vi "TestAFM_Driver_Manager.vi"() -> ()   [LabVIEW 2019]
uses:
  lvsrc/subVIs/AFM API/AFM_Driver_Manager/AFM_Driver_Manager.lvclass
  <vilib>/addons/_JKI Toolkits/Caraya/classes/Test/Test.lvclass
  <vilib>/addons/_JKI Toolkits/Caraya/classes/Assert/Assert.lvclass
  <vilib>/addons/_JKI Toolkits/Caraya/classes/Assert/Assert Equal Value_Variant.vi
  <userlib>/LevyLab/Relay Box/Typedefs/Resistor--enum.ctl
  <vilib>/addons/_JKI Toolkits/Caraya/classes/Assert/Assert True.vi
  <vilib>/addons/_JKI Toolkits/Caraya/classes/Assert/Assert Not Error.vi
panel:
  in  "error in (no error)":errorcluster
  out "error out":errorcluster
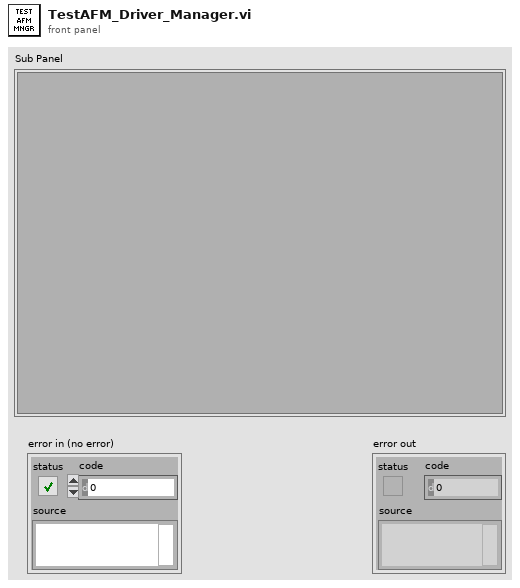
[diagram p1: front panel]
types:
  T1 = typedef "Resistor--enum.ctl" = enum16{"open", "discharge tip", "0 ohms", "100k ohm", "10M ohm", "1G ohm"}
  T2 = cluster{"Name":string, "Litho":cluster{"X":dbl, "Y":dbl, "Speed":dbl, "Voltage":dbl}[], "Set Resistance":T1, "Meta":variant}[]
  T3 = typedef "AFM_Driver_Manager.lvclass/AFM_Driver_Manager.PublicMethods.ctl" = cluster{"Stop Event":refnum<user-event>, "Lithography Data":refnum<user-event>, "Run Lithography":refnum<user-event>, "Background Image":refnum<user-event>, "Abort Notifier":refnum<user-event>}
  T4 = cluster{"VI Refnum":refnum<vi>, "Path":path, "Name":string, "Events":T3}
  T5 = typedef "AFM_Driver_Manager.lvclass/AFM_Driver_Manager.PublicEvents.ctl" = cluster{"Lithography Done":refnum<user-event>}
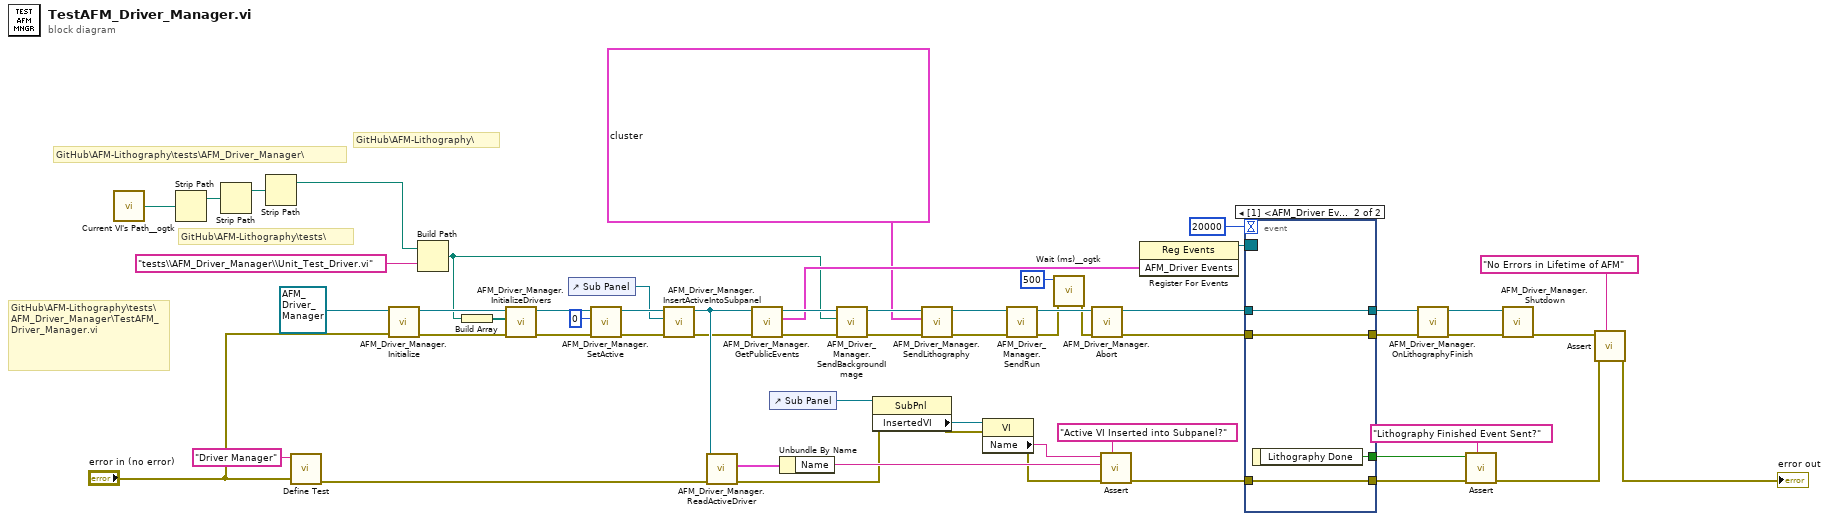
[diagram p0: block diagram]
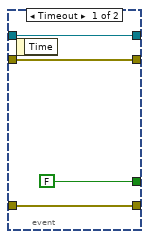
[diagram p2: hidden frame]
diagram:
  # "GitHub\\AFM-Lithography\\tests\\"
  # "GitHub\\AFM-Lithography\\tests\\AFM_Driver_Manager\\"
  # "GitHub\\AFM-Lithography\\"
  # "GitHub\\AFM-Lithography\\tests\\AFM_Driver_Manager\\TestAFM_Driver_Manager.vi"
  n1 = call <userlib>:"Current VI's Path__ogtk.vi"() -> ("Current VI's Path (+ Relative)"=w58:path)  [unwired: 1 in]
  n2 = Strip Path(path=w58) -> (stripped path=w57:path)  [unwired: 1 out]
  n3 = Strip Path(path=w57) -> (stripped path=w56:path)  [unwired: 1 out]
  n4 = Strip Path(path=w56) -> (stripped path=w1:path)  [unwired: 1 out]
  n5 = call <vilib>:"Define Test.vi"("error in (no error)"="error in (no error)", "Label (VI Title)"="Driver Manager") -> ("error out"=w24:errorcluster)  [unwired: 9 in]
  n6 = call "AFM_Driver_Manager.Initialize.vi"("error in (no error)"="error in (no error)", "AFM_Driver_Manager in"=refnum<class "AFM_Driver_Manager.lvclass"> refnum) -> ("error out"=w34:errorcluster, "AFM_Driver_Manager out"=w54:refnum<class "AFM_Driver_Manager.lvclass">)  [unwired: 8 in]
  n7 = Build Path(base path=w1, name or relative path="tests\\AFM_Driver_Manager\\Unit_Test_Driver.vi") -> (appended path=w10:path)
  n8 = Build Array(w10) -> (w31:path[])
  n9 = call "AFM_Driver_Manager.InitializeDrivers.vi"("error in (no error)"=w34, "Paths"=w31, "AFM_Driver_Manager in"=w54) -> ("error out"=w33:errorcluster, "AFM_Driver_Manager out"=w53:refnum<class "AFM_Driver_Manager.lvclass">)  [unwired: 7 in]
  n10 = control-ref of="Sub Panel"() -> (w27:refnum<vi>)
  n11 = call "AFM_Driver_Manager.SetActive.vi"("error in (no error)"=w33, "Active Index"=0, "AFM_Driver_Manager in"=w53) -> ("error out"=w32:errorcluster, "AFM_Driver_Manager out"=w52:refnum<class "AFM_Driver_Manager.lvclass">)  [unwired: 7 in]
  n12 = call "AFM_Driver_Manager.InsertActiveIntoSubpanel.vi"("error in (no error)"=w32, "SubPnl Refnum"=w27, "AFM_Driver_Manager in"=w52) -> ("error out"=w15:errorcluster, "AFM_Driver_Manager out"=w26:refnum<class "AFM_Driver_Manager.lvclass">)  [unwired: 7 in]
  n13 = call "AFM_Driver_Manager.ReadActiveDriver.vi"("error in (no error)"=w24, "AFM_Driver_Manager in"=w26) -> ("error out"=w22:errorcluster, "Active Driver"=w25:T4)  [unwired: 7 in, 1 out]
  n14 = call "AFM_Driver_Manager.GetPublicEvents.vi"("error in (no error)"=w15, "AFM_Driver_Manager in"=w26) -> ("error out"=w49:errorcluster, "AFM_Driver Events"=w35:T5, "AFM_Driver_Manager out"=w50:refnum<class "AFM_Driver_Manager.lvclass">)  [unwired: 7 in]
  n15 = control-ref of="Sub Panel"() -> (w17:refnum<vi>)
  n16 = Unbundle By Name(w25) -> ("Name"=w23:string)
  n17 = call "AFM_Driver_Manager.SendBackgroundImage.vi"("error in (no error)"=w49, "Path"=w10, "AFM_Driver_Manager in"=w50) -> ("error out"=w47:errorcluster, "AFM_Driver_Manager out"=w48:refnum<class "AFM_Driver_Manager.lvclass">)  [unwired: 7 in]
  n18 = property class="SubPnl"(reference=w17, error in=w22) -> (error out=w14:errorcluster, "InsertedVI"=w16:refnum<vi>)  [unwired: 1 out]
  n19 = call "AFM_Driver_Manager.SendLithography.vi"("error in (no error)"=w47, "Lithography Data"=T2 [{"Name"="p0", "Litho"=[{"X"=1.0, "Y"=2.0, "Speed"=3.0, "Voltage"=4.0}], "Set Resistance"=enum."discharge tip", "Meta"=variant}, {"Name"="p1", "Litho"=[{"X"=5.0, "Y"=6.0, "Speed"=7.0, "Voltage"=8.0}], "Set Resistance"=enum."open", "Meta"=variant}], "AFM_Driver_Manager in"=w48) -> ("error out"=w45:errorcluster, "AFM_Driver_Manager out"=w46:refnum<class "AFM_Driver_Manager.lvclass">)  [unwired: 7 in]
  n20 = property class="VI"(reference=w16, error in=w14) -> (error out=w13:errorcluster, "Name"=w12:string)  [unwired: 1 out]
  n21 = call "AFM_Driver_Manager.SendRun.vi"("error in (no error)"=w45, "AFM_Driver_Manager in"=w46) -> ("error out"=w8:errorcluster, "AFM_Driver_Manager out"=w44:refnum<class "AFM_Driver_Manager.lvclass">)  [unwired: 8 in]
  n22 = call <userlib>:"Wait (ms)__ogtk.vi"("error in (no error)"=w8, "milliseconds to wait"=u32 500) -> ("error out"=w9:errorcluster)  [unwired: 8 in, 1 out]
  n23 = call "AFM_Driver_Manager.Abort.vi"("error in (no error)"=w9, "AFM_Driver_Manager in"=w44) -> ("error out"=w38:errorcluster, "AFM_Driver_Manager out"=w40:refnum<class "AFM_Driver_Manager.lvclass">)  [unwired: 8 in]
  n24 = call-poly <vilib>:"Assert.vi"("Label"="Active VI Inserted into Subpanel?" ("Label (VI Title)"), "error in (no error)"=w13, "Y"=w23, "X"=w12) -> ("error out"=w20:errorcluster)  [unwired: 7 in]
  n25 = register-events(w35) -> (reference out=w36:refnum<event-registration>)  [unwired: 2 in, 1 out]
  n26 = event shown="[1] <AFM_Driver Events.Lithography Done>: User Event" {
    selector: w36 -> [_ _]
    dyn-events: _ -> [_ _]
    timeout: 20000 -> [_ _]
    tunnel: [w62 w66] -> w41
    tunnel: w40 -> [w62 w66]
    tunnel: [w61 w65] -> w39
    tunnel: w38 -> [w61 w65]
    tunnel: [FALSE w64] -> w21
    tunnel: w20 -> [w60 w63]
    tunnel: [w60 w63] -> w19
    event Timeout {
      n27 = event-data() -> ()  [unwired: 1 in, 1 out]
    }
    event User Event {
      n28 = event-data() -> ("Lithography Done"=w64:bool)  [unwired: 1 in]
    }
  }
  n29 = call "AFM_Driver_Manager.OnLithographyFinish.vi"("error in (no error)"=w39, "AFM_Driver_Manager in"=w41) -> ("error out"=w42:errorcluster, "AFM_Driver_Manager out"=w43:refnum<class "AFM_Driver_Manager.lvclass">)  [unwired: 8 in]
  n30 = call-poly <vilib>:"Assert.vi"("Label"="Lithography Finished Event Sent?", "error in (no error)"=w19, "True?"=w21) -> ("error out"=w4:errorcluster)  [unwired: 8 in]
  n31 = call "AFM_Driver_Manager.Shutdown.vi"("error in (no error)"=w42, "AFM_Driver_Manager in"=w43) -> ("error out"=w5:errorcluster)  [unwired: 9 in]
  n32 = call-poly <vilib>:"Assert.vi"("Label"="No Errors in Lifetime of AFM", "error in (no error)"=w4, "Not Error?"=w5) -> ("error out"=→"error out":errorcluster)  [unwired: 8 in]
